vi "test-clock-rollover-alg.vi"() -> ()   [LabVIEW 2019]
panel:
  out "Diff":dbl
  out "Loop Count":i32
  in  "Next":bool
  out "Rollover Count":i32
  out "Seconds Out":dbl
  in  "Clock":u32
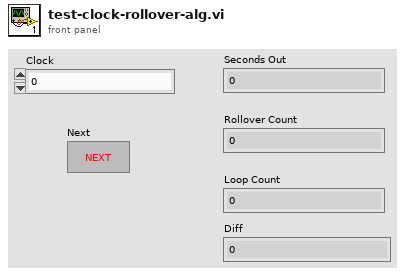
[diagram p1: front panel]
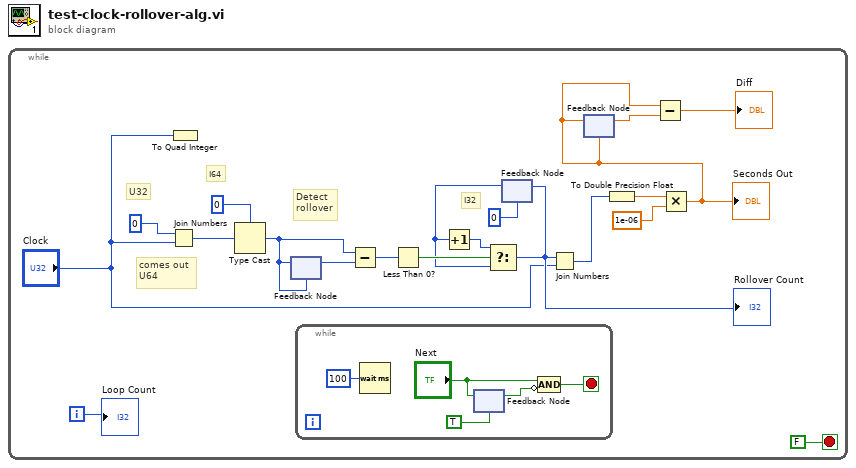
[diagram p0: block diagram]
diagram:
  n1 = while {
    i -> [w5]
    stop <- FALSE stop-if-true
    # "I32"
    # "comes out\nU64"
    # "U32"
    # "I64"
    # "Detect\nrollover"
    n2 = Join Numbers(hi=u32 0, lo="Clock") -> ((hi.lo)=w14:u64)
    n3 = To Quad Integer(1:"Clock") -> ()  [unwired: 1 out]
    n4 = Type Cast(type=i64 0 ("hi"), x=w14) -> (*(type *) &x=w13:i64)
    n5 = feedback #1(w13) -> (w20:i64)
    n6 = feedback-in #1(w13) -> ()
    n7 = while {
      stop <- w22 stop-if-true
      n8 = Wait (ms)(milliseconds to wait=u32 100) -> ()  [unwired: 1 out]
      n9 = feedback-in #2("Next") -> ()
      n10 = feedback #2(TRUE ("Next")) -> (w23:bool)
      n11 = Compound Arithmetic op=AND("Next", invert w23) -> (w22:bool)
    }
    n12 = Subtract(x=w13, y=w20) -> (x-y=w19:i64)
    n13 = Less Than 0?(x=w19) -> (x < 0?=w12:bool)
    n14 = feedback #3(0) -> (w10:i32)
    n15 = Increment(x=w10) -> (x+1=w9:i32)
    n16 = Select(t=w9, s=w12, f=w10) -> (s? t:f=w7:i32)
    "Rollover Count" <- w7
    n17 = feedback-in #3(w7) -> ()
    n18 = Join Numbers(hi=w7, lo="Clock") -> ((hi.lo)=w8:u64)
    n19 = To Double Precision Float(number=w8) -> (double precision float=w17:dbl)
    n20 = Multiply(x=w17, y=1e-06) -> (x*y=w4:dbl)
    "Seconds Out" <- w4
    n21 = feedback-in #4(w4) -> ()
    n22 = feedback #4(w4) -> (w3:dbl)
    n23 = Subtract(x=w4, y=w3) -> (x-y=→"Diff":dbl)
    "Loop Count" <- w5
  }
